vi "DHT12 Read.vi"(8 "Error In":errorcluster, 11 "I2C In":refnum<class "I2C.lvclass">) -> (0 "Error Out":errorcluster, 1 "Humidity":dbl, 2 "Temperature":dbl, 3 "I2C Out":refnum<class "I2C.lvclass">, 4 "Valid":bool)   [LabVIEW 2020, in "lv_dht12.lvlib"]
uses:
  lv_dht12.lvlib
  lv_i2c_hal/I2C/I2C.lvclass
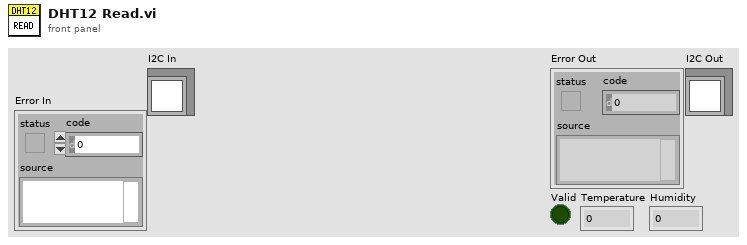
[diagram p1: front panel]
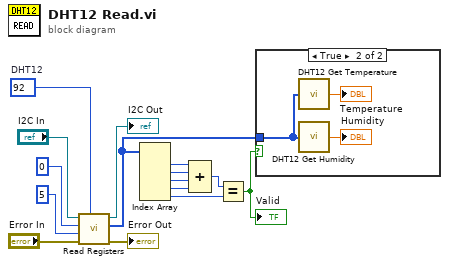
[diagram p0: block diagram]
diagram:
  w15 = u8 92  # DHT12
  n1 = call "Read Registers.vi"("Slave Address"=w15, "Error In"="Error In", "Count"=5, "Register"=u32 0, "I2C In"="I2C In") -> ("Error Out"=→"Error Out":errorcluster, "Values"=w1:u8[], "I2C Out"=→"I2C Out":refnum<class "I2C.lvclass">)  [unwired: 4 in]
  n2 = Index Array(array=w1) -> (element #1=w7:u8, element #2=w6:u8, element #3=w5:u8, element #4=w4:u8, element #5=w3:u8)  [unwired: 5 in]
  n3 = Compound Arithmetic op=ADD(w7, w6, w5, w4) -> (w8:u8)
  n4 = Equal?(x=w8, y=w3) -> (x = y?=w2:bool)
  "Valid" <- w2
  n5 = case shown="True" w2 {
    tunnel: w1 -> [_ w18]
    frame False {
    }
    frame True {
      n6 = call "DHT12 Get Temperature.vi"("Data"=w18) -> ("Temperature"=→"Temperature":dbl)
      n7 = call "DHT12 Get Humidity.vi"("Data"=w18) -> ("Humidity"=→"Humidity":dbl)
    }
  }
